vi "Populating the Asynchronous Call Pool.vi"() -> ()   [LabVIEW 2023]
doc: "<b>Example Description</b>\n\nThis example shows the difference in performance between pre-populating the asynchronous call pool or not. Pre-populating the pool will prevent the Start Asynchronous Call node from needing to switch to the LabVIEW UI thread and create a data space.\n\nWhen running this example, you can see the time it takes to start asynchronous calls is less when the asynchronous call pool was properly pre-populated.\n\n<b>Overview of Asynchronous Call Pool</b>\n\nWhen performing asynchronous calls, an asynchronous call pool of data spaces is automatically created by the Open VI Reference function. By default, the call pool will be sized based on the number of computer cores.\n\nWhen the Start Asynchronous Call node is called, it will attempt to retrieve a data space from the asynchronous call pool. If there are no data spaces available, the Start Asynchronous Call node will automatically create a data space on demand and add it to the pool. This data space creation must be done in the LabVIEW UI thread. The Start Asynchronous Call node will only require the UI thread when it needs to create a data space.\n\nData spaces are automatically returned to the asynchronous call pool differently depending on whether you are performing a call and collect or a call and forget. For the call and collect use case, this is done only after the Wait On Asynchronous Call completes and results have been collected. For the call and forget use case, this is done as soon as the target VI execution completes.\n\nBecause the Start Asynchronous call node can add data spaces to the pool on demand, this can cause short delays when starting a call. These delays can be avoided by using the Populate Asynchronous Call Pool method to create data spaces beforehand."
panel:
  in  "Number of calls":i32=100
  out "Auto Allocate Pool -- Time to start all calls (ms)":u32
  out "Preallocate Pool -- Time to start all calls (ms)":u32
  # "Overview: Demonstrates the use of the  Populate Asynchronous Call Pool method with Asynchronous VI Calls.\nInstructions:\nRun the VI. Observe the benchmark values below. See the block diagram for more information."
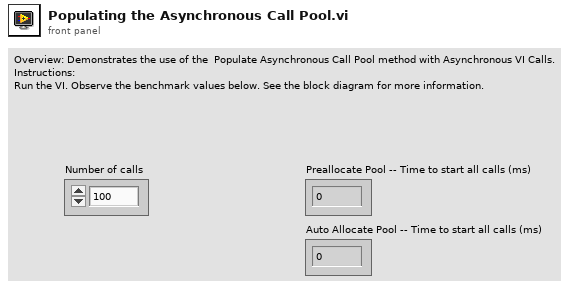
[diagram p1: front panel]
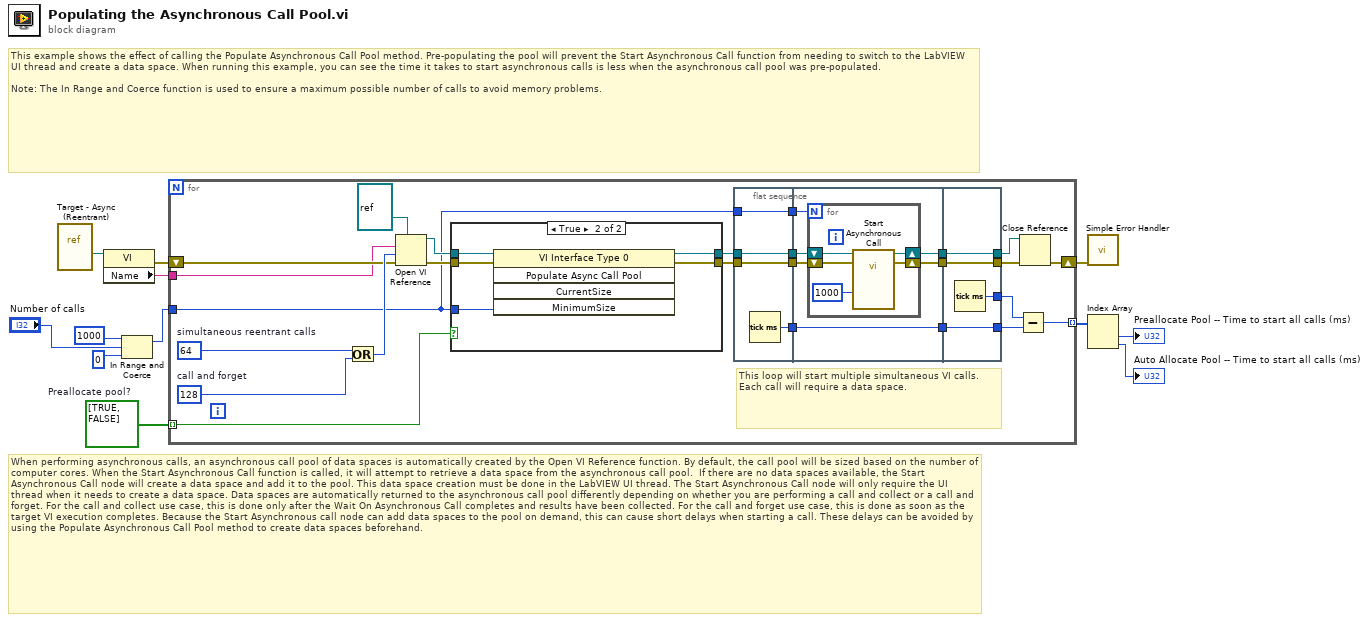
[diagram p0: block diagram]
diagram:
  w12 = bool[] [TRUE, FALSE]  # Preallocate pool?
  # "When performing asynchronous calls, an asynchronous call pool of data spaces is automatically created by the Open VI Reference function. By default, the call pool will be sized based on the number of computer cores. When the Start Asynchronous Call function is called, it will attempt to retrieve a data space from the asynchronous call pool.  If there are no data spaces available, the Start Asynchronous Call node will create a data space and add it to the pool. This data space creation must be done in the LabVIEW UI thread. The Start Asynchronous Call node will only require the UI thread when it needs to create a data space. Data spaces are automatically returned to the asynchronous call pool differently depending on whether you are performing a call and collect or a call and forget. For the call and collect use case, this is done only after the Wait On Asynchronous Call completes and results have been collected. For the call and forget use case, this is done as soon as the target VI execution completes. Because the Start Asynchronous call node can add data spaces to the pool on demand, this can cause short delays when starting a call. These delays can be avoided by using the Populate Asynchronous Call Pool method to create data spaces beforehand."
  # "This example shows the effect of calling the Populate Asynchronous Call Pool method. Pre-populating the pool will prevent the Start Asynchronous Call function from needing to switch to the LabVIEW UI thread and create a data space. When running this example, you can see the time it takes to start asynchronous calls is less when the asynchronous call pool was pre-populated.\n\nNote: The In Range and Coerce function is used to ensure a maximum possible number of calls to avoid memory problems."
  n1 = vi-ref "Target - Async (Reentrant).vi"() -> (w3:refnum<vi>)
  n2 = property class="VI"(reference=w3) -> (error out=w2:errorcluster, "Name"=w1:string)  [unwired: 1 in, 1 out]
  n3 = In Range and Coerce(upper limit=1000 ("y"), x="Number of calls", lower limit=0) -> (coerced(x)=w6:i32)  [unwired: 1 out]
  n4 = for {
    tunnel: [w19] -> w11 mode=indexing
    tunnel: w12 -> [w18] mode=indexing
    tunnel: w6 -> [w17]
    shift-right: [w28] -> w4
    shift-left: w2 -> [w14]
    tunnel: w1 -> [w13]
    w15 = 64  # simultaneous reentrant calls
    w27 = 128  # call and forget
    # "This loop will start multiple simultaneous VI calls. Each call will require a data space."
    n5 = Or(x=w15, y=w27) -> (x .or. y?=w26:i32)
    n6 = Open VI Reference(type specifier VI Refnum (for type only)=refnum<vi> refnum, vi path=w13, options=w26, error in (no error)=w14) -> (vi reference=w25:refnum<vi>, error out=w24:errorcluster)  [unwired: 2 in]
    n7 = case shown="True" w18 {
      tunnel: w25 -> [w39 w44]
      tunnel: w24 -> [w38 w43]
      tunnel: [w39 w42] -> w23
      tunnel: [w38 w41] -> w22
      tunnel: w17 -> [_ w40]
      frame False {
      }
      frame True {
        n8 = invoke class="VI Interface Type 0" method="Populate Async Call Pool"(reference=w44, error in=w43, "MinimumSize"=w40) -> (reference out=w42:refnum<vi>, error out=w41:errorcluster)  [unwired: 2 in, 3 out]
      }
    }
    n9 = flat-sequence {
      tunnel: w22 -> [w47]
      tunnel: w23 -> [w48]
      tunnel: [w48] -> w37
      tunnel: [w47] -> w36
      tunnel: [w46] -> w35
      tunnel: w17 -> [w45]
      tunnel: [w45] -> w16
      tunnel: [w54] -> w34
      tunnel: [w53] -> w33
      tunnel: w37 -> [w52]
      tunnel: w36 -> [w51]
      tunnel: [w50] -> w32
      tunnel: w35 -> [w50]
      tunnel: w16 -> [w49]
      tunnel: [w62] -> w29
      tunnel: [w63] -> w30
      tunnel: w34 -> [w63]
      tunnel: w33 -> [w62]
      tunnel: [w61] -> w21
      tunnel: [w60] -> w20
      tunnel: w32 -> [w60]
      frame #0 {
        n10 = Tick Count (ms)() -> (millisecond timer value=w46:u32)
      }
      frame #1 {
        n11 = for {
          N: w49 -> [_]
          shift-right: [w59] -> w54
          shift-left: w51 -> [w56]
          shift-right: [w58] -> w53
          shift-left: w52 -> [w57]
          n12 = call-by-ref "Start Asynchronous Call"(reference=w57, error in=w56, "Wait (Milliseconds)"=u32 1000) -> (reference out=w58:refnum<vi>, error out=w59:errorcluster)  [unwired: 10 in, 1 out]
        }
      }
      frame #2 {
        n13 = Tick Count (ms)() -> (millisecond timer value=w61:u32)
      }
    }
    n14 = Subtract(x=w21, y=w20) -> (x-y=w19:u32)
    n15 = Close Reference(reference=w29, error in (no error)=w30) -> (error out=w28:errorcluster)
  }
  n16 = call <vilib>:"Simple Error Handler.vi"("error in (no error)"=w4) -> ()  [unwired: 4 in, 5 out]
  n17 = Index Array(array=w11) -> (element #1=→"Preallocate Pool -- Time to start all calls (ms)":u32, element #2=→"Auto Allocate Pool -- Time to start all calls (ms)":u32)  [unwired: 2 in]
